vi "Module Identities.vi"(8 "error in (no error)":errorcluster, 11 "System Config Module in":refnum<class "System Config Module.lvclass">) -> (0 "error out":errorcluster, 2 "Identities":refnum<class "Identity.lvclass">[](array[class]), 3 "System Config Module out":refnum<class "System Config Module.lvclass">)   [LabVIEW 2020, in "Volatus.lvlib" / "System Config Module.lvclass"]
uses:
  System Config Module.lvclass
  Identity/Identity.lvclass
  System Config Module.lvclass/System Config Module.ctl
  System Config Identity/System Config Identity.lvclass
  C:/dev/lv20CE/relink/lv-volatus/Volatus/System Config Identity/System Config Identity.lvclass
  C:/dev/lv20CE/relink/lv-volatus/Volatus/Identity/Identity.lvclass
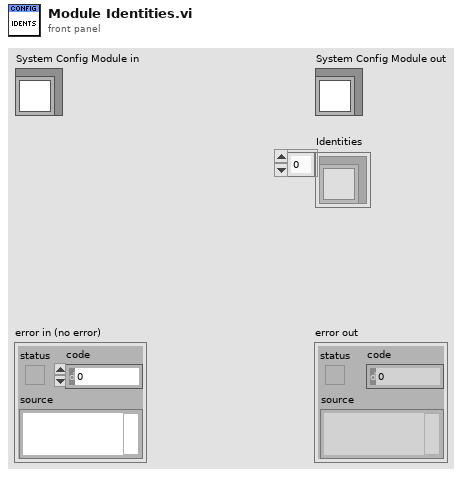
[diagram p1: front panel]
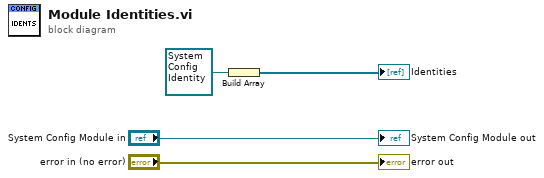
[diagram p0: block diagram]
diagram:
  n1 = Build Array(refnum<class "System Config Identity.lvclass"> refnum ("Volatus:System Config Identity.lvclass")) -> (→"Identities":refnum<class "System Config Identity.lvclass">[])
  "error out" <- "error in (no error)"
  "System Config Module out" <- "System Config Module in"
